vi "ALU (SubVI).vi"(4 "Output Array  2":dbl[](array[numeric]), 6 "Ex.AddressIn2":fxp<+,16,16>, 7 "DataMemory/Fxp in":dbl[](array[numeric]), 8 "Input Array":dbl[](array[numeric]), 9 "Ex.AddressIn1":fxp<+,16,16>, 10 "WB.Command in":T1, 11 "WB.AddressOut":fxp<+,16,16>) -> (0 "output array":dbl[](array[numeric]), 1 "currrent output":dbl, 2 "DataMemory/Fxp out":dbl[](array[numeric]), 3 "WB.Command out":T1=enum."None")   [LabVIEW 2016]
uses:
  Z:/original_project/CodeConverter/Controls/WB.Operation.ctl
  Z:/original_project/CodeConverter/SoftCoreCodeConverter.lvlib
panel:
  out "DataMemory/out":dbl[](array[numeric])
  in  "WB.AddressOut":fxp<+,16,16>
  in  "Ex.AddressIn1":fxp<+,16,16>
  in  "Ex.AddressIn2":fxp<+,16,16>
  in  "DataMemory/In":dbl[](array[numeric])
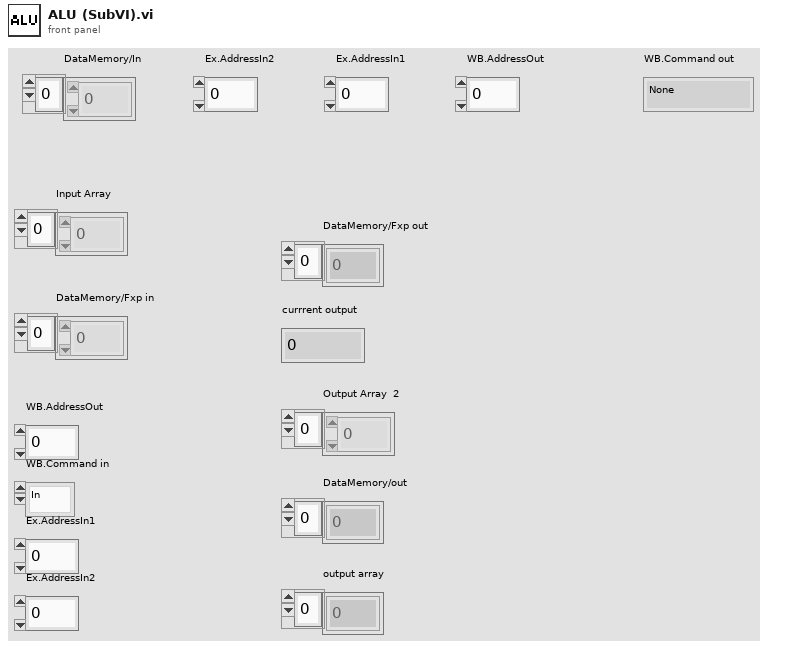
[diagram p1: front panel]
types:
  T1 = typedef "SoftCoreCodeConverter.lvlib/WB.Operation.ctl" = enum8{"In", "Out", "Mov", "Add", "Sub", "Mul", "Div", "None", "Sqr", "Sin", "Cos", "Sgl2Dbl", "Dbl2Int", "Int2Dbl", "Mlookup", "Dbl2Sgl", "G_IsPOS", "G_IsNEG", "G_IsNULL", "G_IsNNULL", "G_IsNAN", "G_IsNNAN", "G_IsIFTY", "G_IsNIFTY", "reserved_0", "reserved_1", "reserved_2", "reserved_3", "reserved_4", "reserved_5", "reserved_6", "reserved_7"}
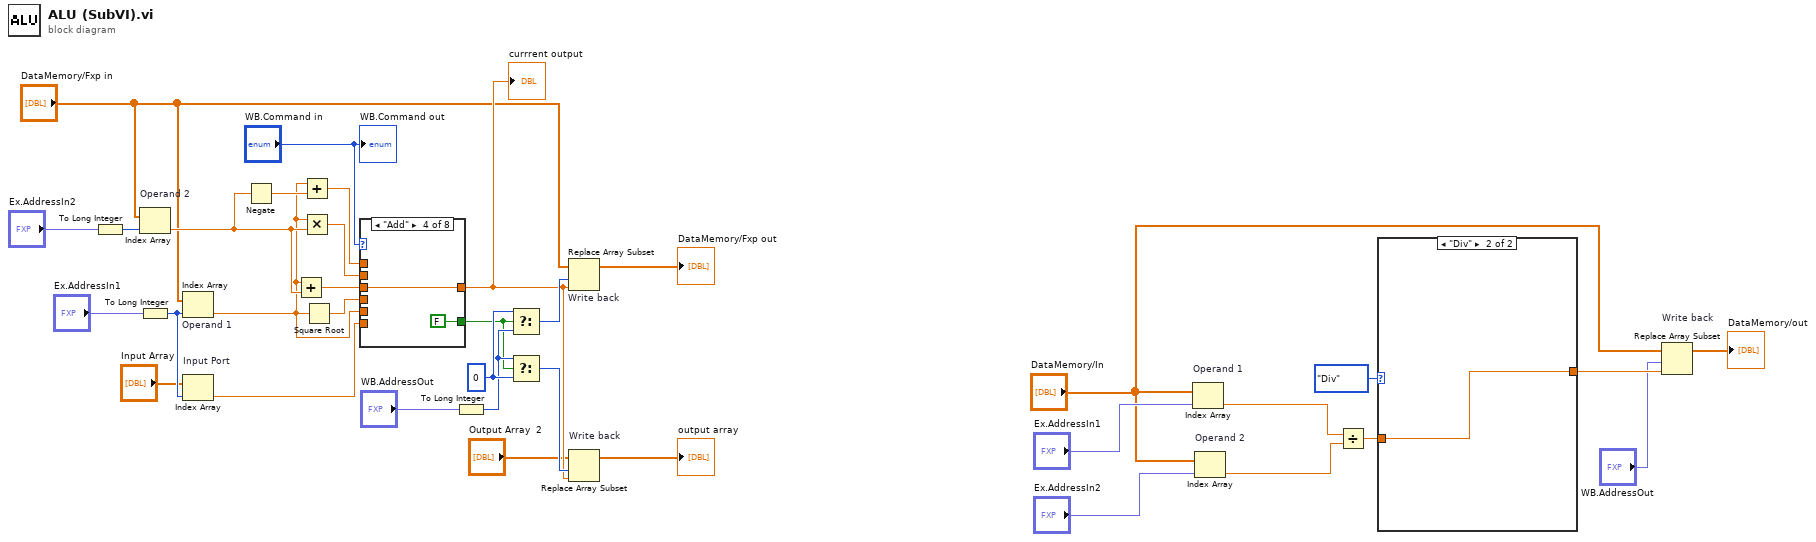
[diagram p0: block diagram]
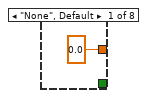
[diagram p3: hidden frame]
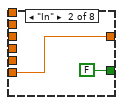
[diagram p4: hidden frame]
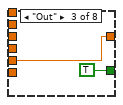
[diagram p5: hidden frame]
diagram:
  w20 = 0 ("f")
  n1 = To Long Integer(number="Ex.AddressIn2") -> (32bit integer=w31:i32)
  n2 = Index Array "Operand 2"(array="DataMemory/Fxp in", index=w31) -> (element=w33:dbl)
  n3 = To Long Integer(number="Ex.AddressIn1") -> (32bit integer=w24:i32)
  n4 = Index Array "Operand 1"(array="DataMemory/Fxp in", index=w24) -> (element=w21:dbl)
  n5 = Index Array "Input Port"(array="Input Array", index=w24) -> (element=w23:dbl)
  n6 = Negate(x=w33) -> (-x=w30:dbl)
  n7 = Add(x=w21, y=w33) -> (x+y=w32:dbl)
  n8 = Add(x=w21, y=w30) -> (x+y=w29:dbl)
  n9 = Multiply(x=w21, y=w33) -> (x*y=w28:dbl)
  n10 = Square Root(x=w21) -> (sqrt(x)=w34:dbl)
  n11 = case shown="\"Add\"" "WB.Command in" {
    tunnel: w28 -> [_ _ _ _ w43 _ _ _]
    tunnel: [0.0 w38 w39 w42 w43 w44 w45 w46] -> w15
    tunnel: w29 -> [_ _ _ _ _ w44 _ _]
    tunnel: w32 -> [_ _ _ w42 _ _ _ _]
    tunnel: w21 -> [_ _ w39 _ _ _ _ w46]
    tunnel: w34 -> [_ _ _ _ _ _ w45 _]
    tunnel: w23 -> [_ w38 _ _ _ _ _ _]
    tunnel: [_ FALSE TRUE FALSE _ _ _ _] -> w18
    frame "None", Default {
    }
    frame "In" {
    }
    frame "Out" {
    }
    frame "Add" {
    }
    frame "Mul" {
    }
    frame "Sub" {
    }
    frame "Sqr" {
    }
    frame "Mov" {
    }
  }
  "currrent output" <- w15
  n12 = To Long Integer(number="WB.AddressOut") -> (32bit integer=w19:i32)
  n13 = Select(t=w20, s=w18, f=w19) -> (s? t:f=w17:i32)
  n14 = Select(t=w19, s=w18, f=w20) -> (s? t:f=w16:i32)
  n15 = Replace Array Subset "Write back"(array="DataMemory/Fxp in", new element=w15, index=w17) -> (→"DataMemory/Fxp out":dbl[])
  n16 = Replace Array Subset "Write back"(array="Output Array  2", new element=w15, index=w16) -> (→"output array":dbl[])
  n17 = Index Array "Operand 1"(array="DataMemory/In", index="Ex.AddressIn1") -> (element=w10:dbl)
  n18 = Index Array "Operand 2"(array="DataMemory/In", index="Ex.AddressIn2") -> (element=w11:dbl)
  n19 = Divide(x=w10, y=w11) -> (x/y=w9:dbl)
  n20 = case shown="\"Div\"" WB.Operation."Div" ("WB.Command in") {
    tunnel: w9 -> [_ w47]
    tunnel: [_ w47] -> w6
    frame "In", Default {
    }
    frame "Div" {
    }
  }
  n21 = Replace Array Subset "Write back"(array="DataMemory/In", new element=w6, index="WB.AddressOut") -> (→"DataMemory/out":dbl[])
  "WB.Command out" <- "WB.Command in"
